vi "PH_GetRates_SubVI.vi"(7 "APD num":enum16{"NA", "APD1", "APD2", "APD1+2"}(ring), 8 "PH_Settings_Params":T2={"SyncDiv"=1, "DeviceIndex"=0, "CFD0 level"=50, "CFD0 zero X"=10, "CFD1 level"=50, "CFD1 zero X"=10, "Range No."=0, "StopOnOverflow"=FALSE, "AcqTime (ms)"=0.0} {"Range No." min=0 max=5 step=1; "CFD1 zero X" min=0 max=40 step=1; "CFD1 level" min=0 max=400 step=1; "CFD0 zero X" min=-1300 max=400 step=10; "CFD0 level" min=-1300 max=400 step=10; "SyncDiv" min=1 max=8 step=1}, 9 "PH_Init_Data":T1, 10 "Stop PD Ref":refnum<vi>, 11 "PD 1D Spectrum Ref":refnum<vi>) -> (2 "APD1+2":dbl[][](array[numeric]))   [LabVIEW 2019]
panel:
  out "Empty":dbl[](array[numeric])
  out "APD2":dbl[](array[numeric])
  out "APD1":dbl[](array[numeric])
  out "PD 1D Spectrum":dbl[][](graph)
  out "Waveform Graph 2":dbl[][](graph)
  in  "Stop PD":bool
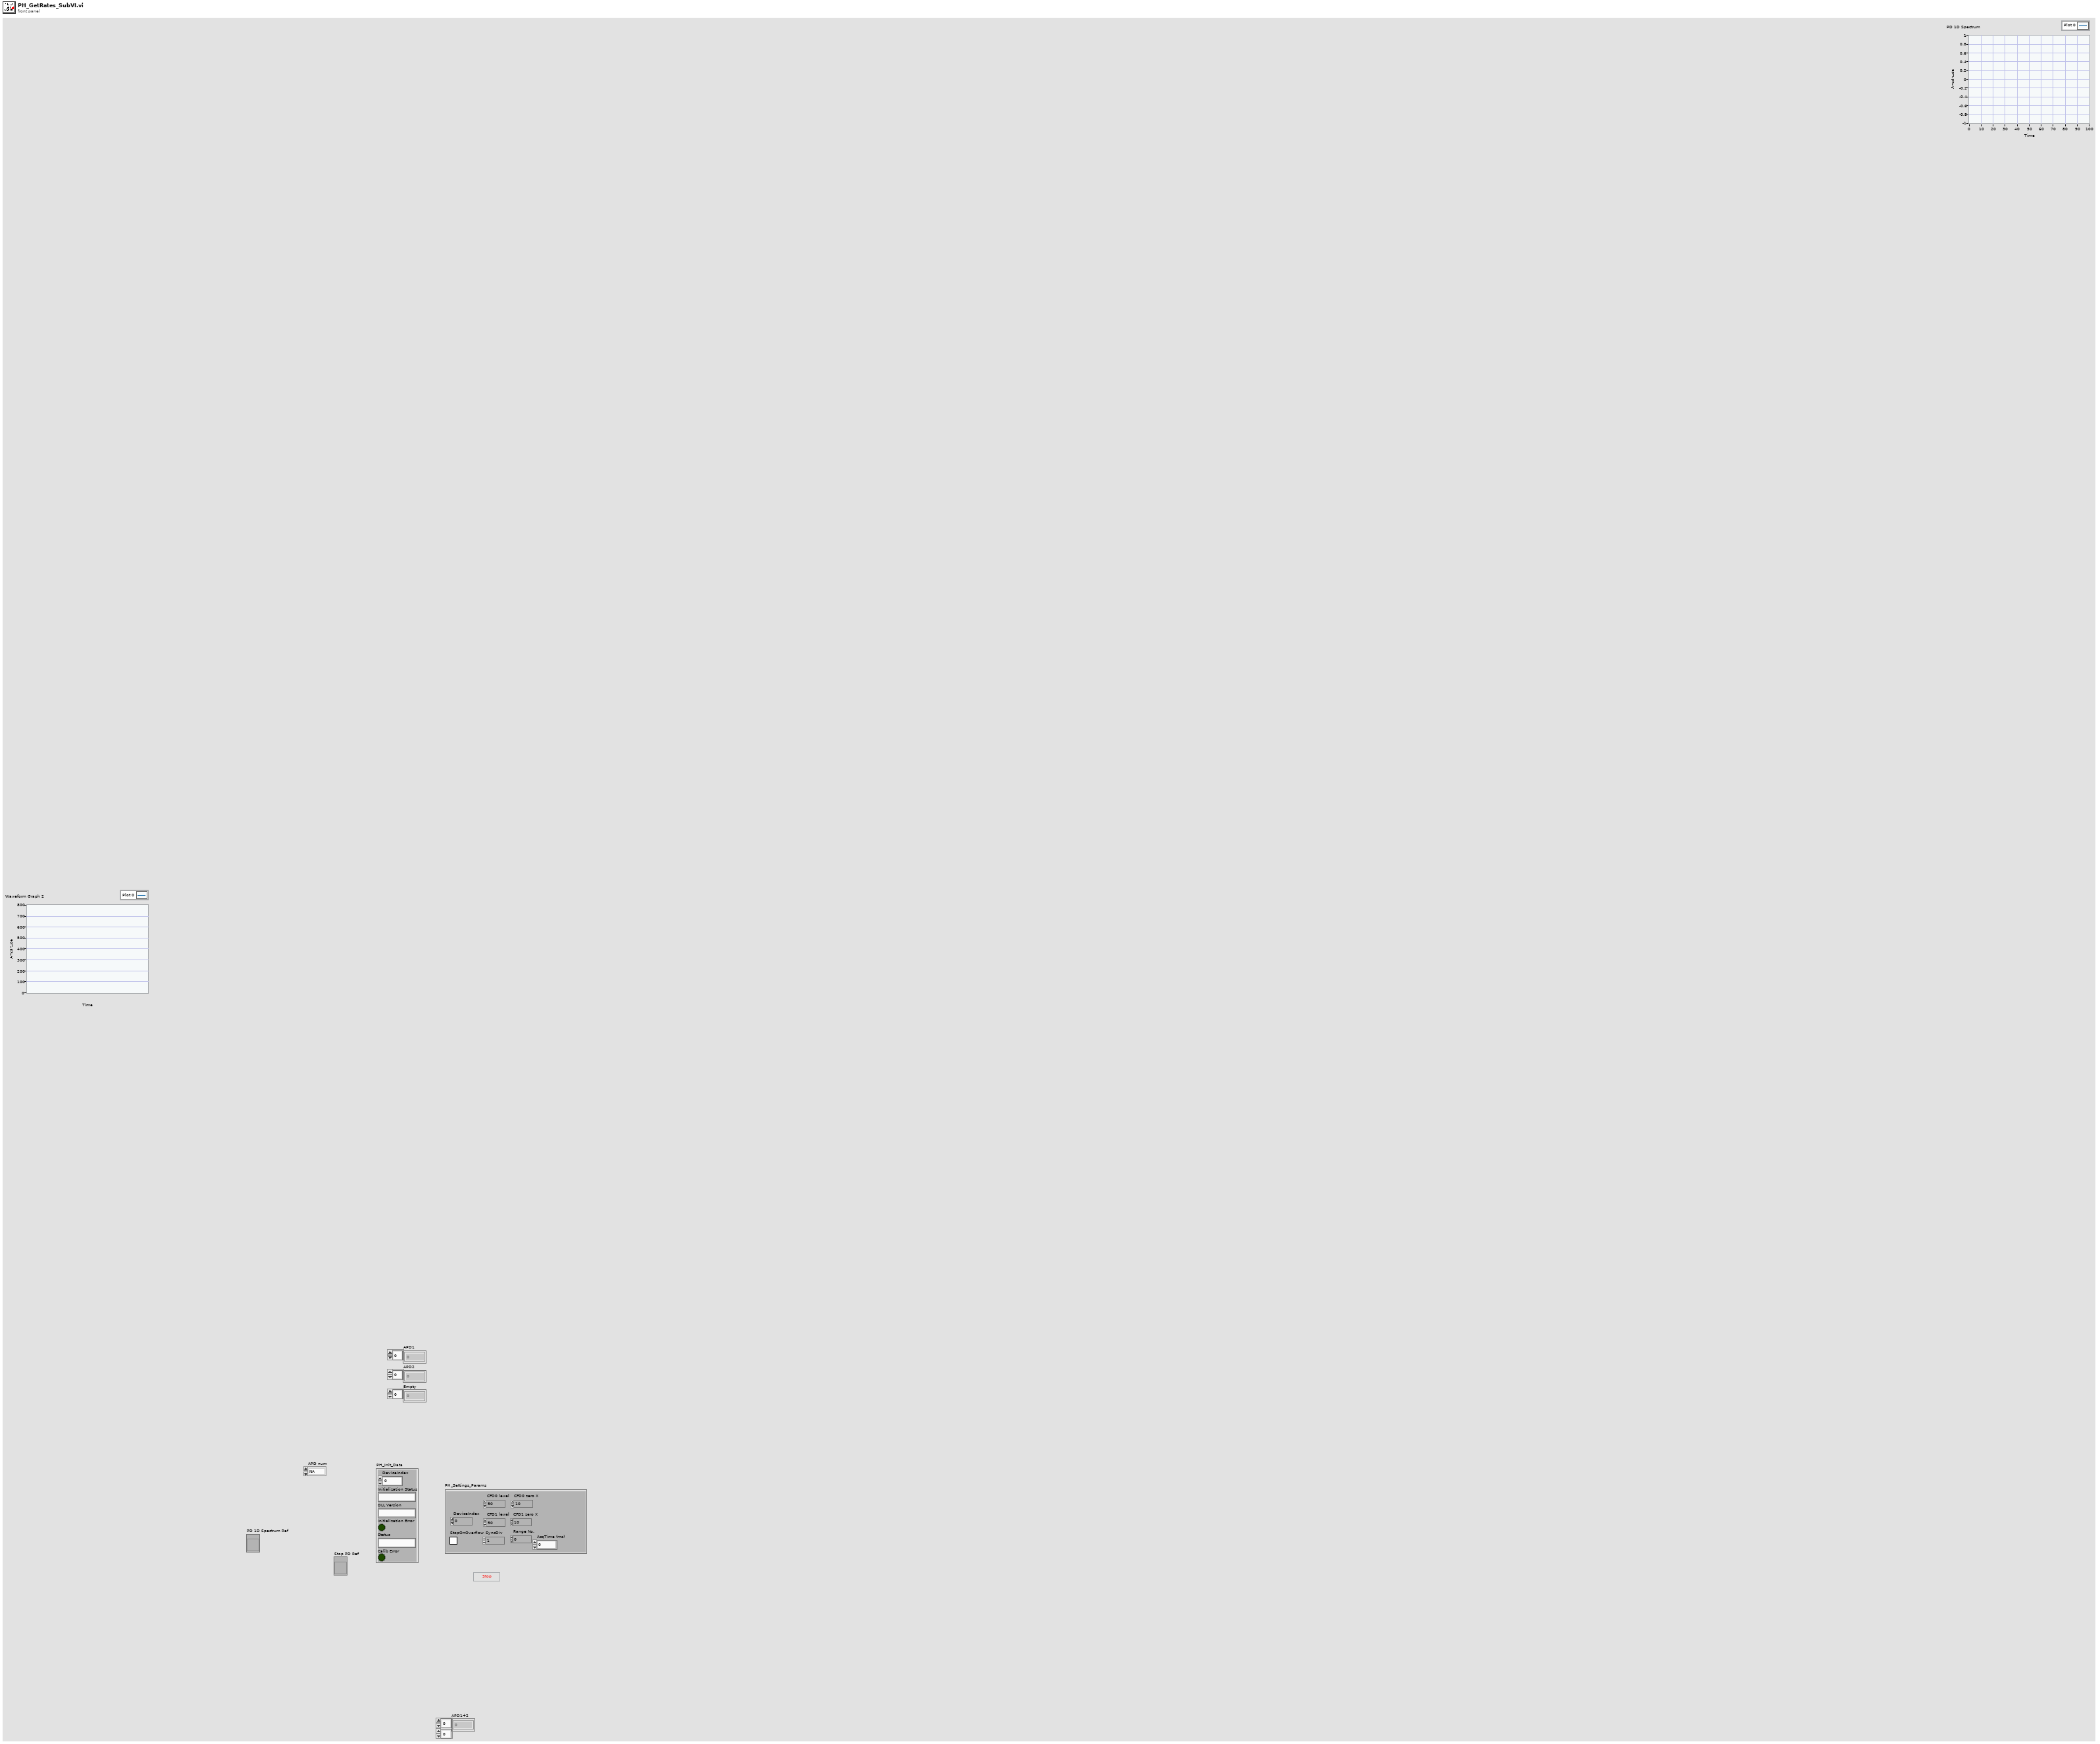
[diagram p1: front panel]
types:
  T1 = cluster{"Deviceindex":i32, "Initialization Status":string, "DLL Version":string, "Initialization Error":bool, "Status":string, "Calib Error":bool}
  T2 = cluster{"SyncDiv":i32, "DeviceIndex":i32, "CFD0 level":i32, "CFD0 zero X":i32, "CFD1 level":i32, "CFD1 zero X":i32, "Range No.":i32, "StopOnOverflow":bool, "AcqTime (ms)":dbl}
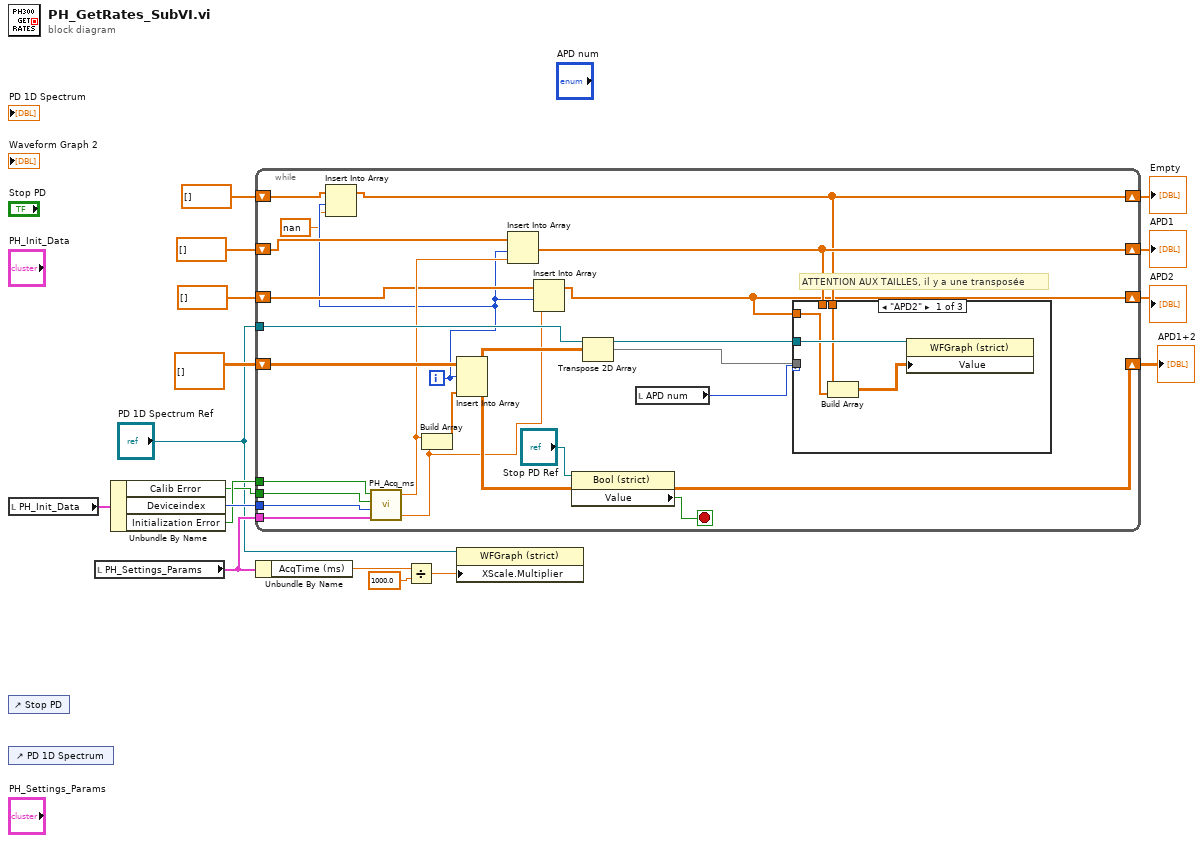
[diagram p0: block diagram]
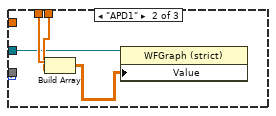
[diagram p2: hidden frame]
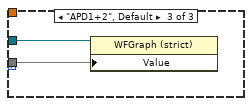
[diagram p3: hidden frame]
diagram:
  n1 = local read "PH_Init_Data"() -> (w17:T1)
  n2 = control-ref of="Stop PD"() -> ()  [unwired: 1 out]
  n3 = control-ref of="PD 1D Spectrum"() -> ()  [unwired: 1 out]
  n4 = local read "PH_Settings_Params"() -> (w11:T2)
  n5 = Unbundle By Name(w17) -> ("Calib Error"=w14:bool, "Deviceindex"=w16:i32, "Initialization Error"=w15:bool)
  n6 = while {
    tunnel: w16 -> [w39]
    tunnel: w15 -> [w38]
    tunnel: w14 -> [w37]
    tunnel: w11 -> [w33]
    shift-right: [w34] -> w12
    shift-left: dbl[][] [] -> [w36]
    tunnel: "PD 1D Spectrum Ref" -> [w31]
    shift-right: [w20] -> w4
    shift-left: dbl[] [] -> [w28]
    shift-right: [w18] -> w3
    shift-left: dbl[] [] -> [w26]
    shift-right: [w19] -> w1
    shift-left: dbl[] [] -> [w24]
    i -> [w23]
    stop <- w30 stop-if-true
    # "ATTENTION AUX TAILLES, il y a une transposée"
    n7 = Insert Into Array(array=w24, index=w23, new element=nan) -> (w19:dbl[])
    n8 = call "PH_Acq_ms.vi"("PH_Settings_Params"=w33, "Deviceindex"=w39, "Calib Error"=w37, "Initialization Error"=w38) -> ("CH1MeanRate"=w25:dbl, "SyncMeanRate"=w27:dbl)  [unwired: 1 out]
    n9 = Build Array(w27, w25) -> (w35:dbl[])
    n10 = Insert Into Array(array=w36, index (row)=w23, new element=w35) -> (w34:dbl[][])  [unwired: 1 in]
    n11 = Insert Into Array(array=w28, index=w23, new element=w27) -> (w20:dbl[])
    n12 = Insert Into Array(array=w26, index=w23, new element=w25) -> (w18:dbl[])
    n13 = property class="Bool (strict)"(reference="Stop PD Ref") -> ("Value"=w30:bool)  [unwired: 1 in, 2 out]
    n14 = Transpose 2D Array(2D array=w34) -> (transposed array=w32:dbl[][])
    n15 = local read "APD num"() -> (w21:enum16{"NA", "APD1", "APD2", "APD1+2"})
    n16 = case shown="\"APD2\"" w21 {
      tunnel: w32 -> [_ _ w49]
      tunnel: w31 -> [w43 w45 w48]
      tunnel: w20 -> [_ w47 _]
      tunnel: w19 -> [w42 w46 _]
      tunnel: w18 -> [w41 _ _]
      frame "APD2" {
        n17 = Build Array(w42, w41) -> (w40:dbl[][])
        n18 = property class="WFGraph (strict)"(reference=w43, "Value"=w40) -> ()  [unwired: 1 in, 2 out]
      }
      frame "APD1" {
        n19 = Build Array(w47, w46) -> (w44:dbl[][])
        n20 = property class="WFGraph (strict)"(reference=w45, "Value"=w44) -> ()  [unwired: 1 in, 2 out]
      }
      frame "APD1+2", Default {
        n21 = property class="WFGraph (strict)"(reference=w48, "Value"=w49) -> ()  [unwired: 1 in, 2 out]
      }
    }
  }
  "APD1+2" <- w12
  "APD1" <- w4
  "APD2" <- w3
  "Empty" <- w1
  n22 = Unbundle By Name(w11) -> ("AcqTime (ms)"=w9:dbl)
  n23 = Divide(x=w9, y=1000.0) -> (x/y=w7:dbl)
  n24 = property class="WFGraph (strict)"(reference="PD 1D Spectrum Ref", "XScale.Multiplier"=w7) -> ()  [unwired: 1 in, 2 out]
